vi "PythonBoolean.vi"(11 "Python Boolean as String":string) -> (3 "Boolean":bool)   [LabVIEW 2015]
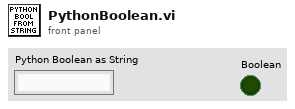
[diagram p1: front panel]
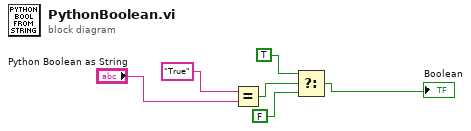
[diagram p0: block diagram]
diagram:
  n1 = Equal?(x="True", y="Python Boolean as String") -> (x = y?=w2:bool)
  n2 = Select(t=TRUE, s=w2, f=FALSE) -> (s? t:f=→"Boolean":bool)
